vi "test_read_SV.vi"() -> ()   [LabVIEW 2017]
panel:
  out "error out 2":errorcluster
  out "error out":errorcluster
  in  "stop":bool
  out "Theta":dbl
  out "Distance":dbl
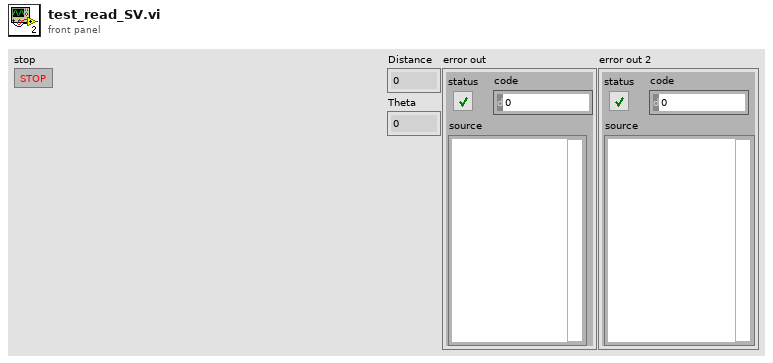
[diagram p1: front panel]
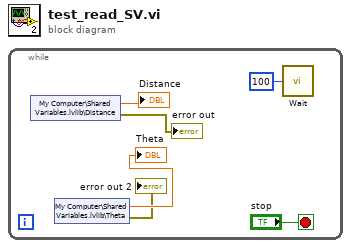
[diagram p0: block diagram]
diagram:
  n1 = while {
    stop <- "stop" stop-if-true
    n2 = shared-variable "My Computer\\Shared Variables.lvlib\\Distance"() -> (→"Distance":dbl, error out=→"error out":errorcluster)  [unwired: 1 in]
    n3 = shared-variable "My Computer\\Shared Variables.lvlib\\Theta"() -> (→"Theta":dbl, error out=→"error out 2":errorcluster)  [unwired: 1 in]
    n4 = call "Wait"("Count(mSec)"=u32 100) -> ()  [unwired: 1 out]
  }
